vi "test_se_main_sid.vi"() -> ()   [LabVIEW 2016]
uses:
  <vilib>/rvi/DesktopExecutionNode/Execution/niFpgaDEN_Execute.vi
  <vilib>/rvi/DesktopExecutionNode/DesktopExecutionNode.xnode
panel:
  in  "se.sid.idParams":T1
  out "prbsSignal":T2(array[cluster])
  out "positionGraph":dbl[][](graph)
  out "positionGraph 2":dbl[][](graph)
  in  "scanTurnOnTime":i32=500
  out "itcSIDOutput":bool[](array[boolean])
  out "sidRepetition":u16[](array[numeric])
  out "sidRunning":bool[](array[boolean])
  out "positionSID":T3(array[cluster]) {"outputInt"."x" format="%.17g"; "outputInt"."y" format="%.17g"}
  out "position":T4(array[cluster]) {"outputInt"."x" format="%.16g"; "outputInt"."y" format="%.16g"}
  in  "se.sid.axisXnotY":bool=TRUE
  in  "sidOnTime":i32=6000
  in  "se.p.clocks":T5={"outputRate"=4, "fastDecFactor"=0, "outWaveSizeFast"=128, "pplUpsampling"=0, "numLines"=16, "se.p.fastInvDec"=0.0, "se.p.slowUpStep"=0.0, "se.p.outWaveSizeSlow"=128, "blankingMax"=6000000, "se.p.fastBlanking"={"startFwd"=0, "endFwd"=0, "startBwd"=0, "endBwd"=0, "disableBlanking"=TRUE, "useCoarseCounter"=FALSE}}
  in  "se.mot.p.target":cluster{"x":fxp<+/-,16,1>, "y":fxp<+/-,16,1>}[](array[cluster])=[{"x"=0.20001220703125, "y"=0.20001220703125}]
  in  "outputParams":T6={"se.p.scanOffsets"={"x"=0.0, "y"=0.0}, "se.p.transformMatrix"={"a"=1.0, "b"=0.0, "c"=0.0, "d"=1.0}, "se.p.scanSize"={"fastScanSize"=0.399993896484375, "slowScanSize"=0.399993896484375, "invertSlowAxis"=FALSE}}
  in  "se.p.modes":T7
  in  "se.mot.p.clocks":T8={"moveToDecFactor"=9, "moveToWaveSize"=128, "se.mot.p.invDec"=0.0}
  out "simulationProgressDone":dbl(slide)=0.9999166666666667 scale=0.0..1.0
  in  "simulationTime (ticks)":i32=12000
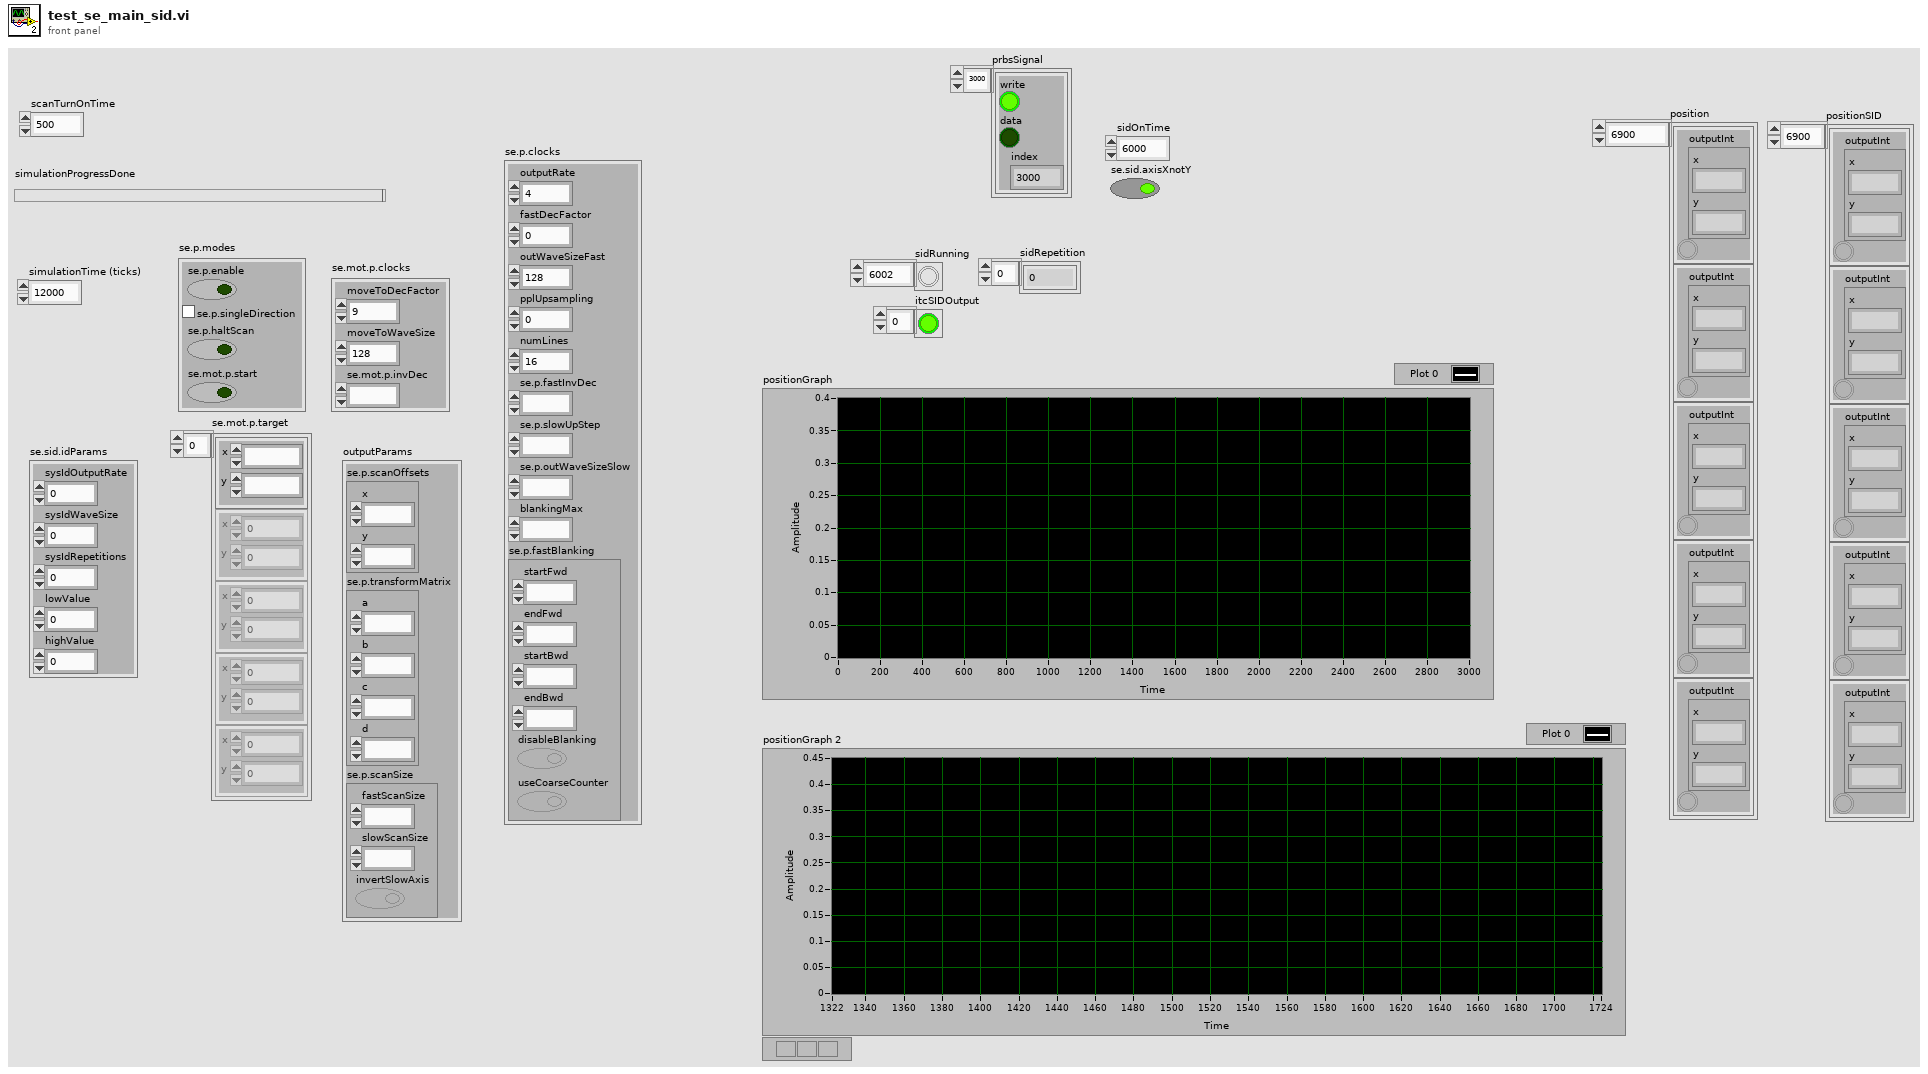
[diagram p1: front panel]
types:
  T1 = cluster{"sysIdOutputRate":u16, "sysIdWaveSize":u16, "sysIdRepetitions":u16, "lowValue":fxp<+/-,16,1>, "highValue":fxp<+/-,16,1>}
  T2 = cluster{"write":bool, "data":bool, "index":u16}[]
  T3 = cluster{"outputInt":cluster{"sid.o.height":fxp<+/-,28,1>, "sid.o.height":fxp<+/-,28,1>}, bool}[]
  T4 = cluster{"outputInt":cluster{"y":fxp<+/-,16,1>, "y":fxp<+/-,16,1>}, bool}[]
  T5 = cluster{"outputRate":u16, "fastDecFactor":u16, "outWaveSizeFast":u16, "pplUpsampling":u16, "numLines":u16, "se.p.fastInvDec":fxp<+,22,0>, "se.p.slowUpStep":fxp<+,28,0>, "se.p.outWaveSizeSlow":u16, "blankingMax":u32, "se.p.fastBlanking":cluster{"startFwd":u32, "endFwd":u32, "startBwd":u32, "endBwd":u32, "disableBlanking":bool, "useCoarseCounter":bool}}
  T6 = cluster{"se.p.scanOffsets":cluster{"x":fxp<+/-,16,1>, "y":fxp<+/-,16,1>}, "se.p.transformMatrix":cluster{"a":fxp<+/-,18,2>, "b":fxp<+/-,18,2>, "c":fxp<+/-,18,2>, "d":fxp<+/-,18,2>}, "se.p.scanSize":cluster{"fastScanSize":fxp<+,17,1>, "slowScanSize":fxp<+,17,1>, "invertSlowAxis":bool}}
  T7 = cluster{"se.p.enable":bool, "se.p.singleDirection":bool, "se.p.haltScan":bool, "se.mot.p.start":bool}
  T8 = cluster{"moveToDecFactor":u16, "moveToWaveSize":u16, "se.mot.p.invDec":fxp<+,16,0>}
  T9 = cluster{"a":fxp<+/-,18,2>, "b":fxp<+/-,18,2>, "c":fxp<+/-,18,2>, "d":fxp<+/-,18,2>}
  T10 = cluster{"fastScanSize":fxp<+,17,1>, "slowScanSize":fxp<+,17,1>, "invertSlowAxis":bool}
  T11 = cluster{"outputInt":cluster{"y":fxp<+/-,16,1>, "y":fxp<+/-,16,1>}, bool}
  T12 = cluster{"outputInt":cluster{"sid.o.height":fxp<+/-,28,1>, "sid.o.height":fxp<+/-,28,1>}, bool}
  T13 = cluster{"sid.o.height":fxp<+/-,28,1>, "sid.o.height":fxp<+/-,28,1>}
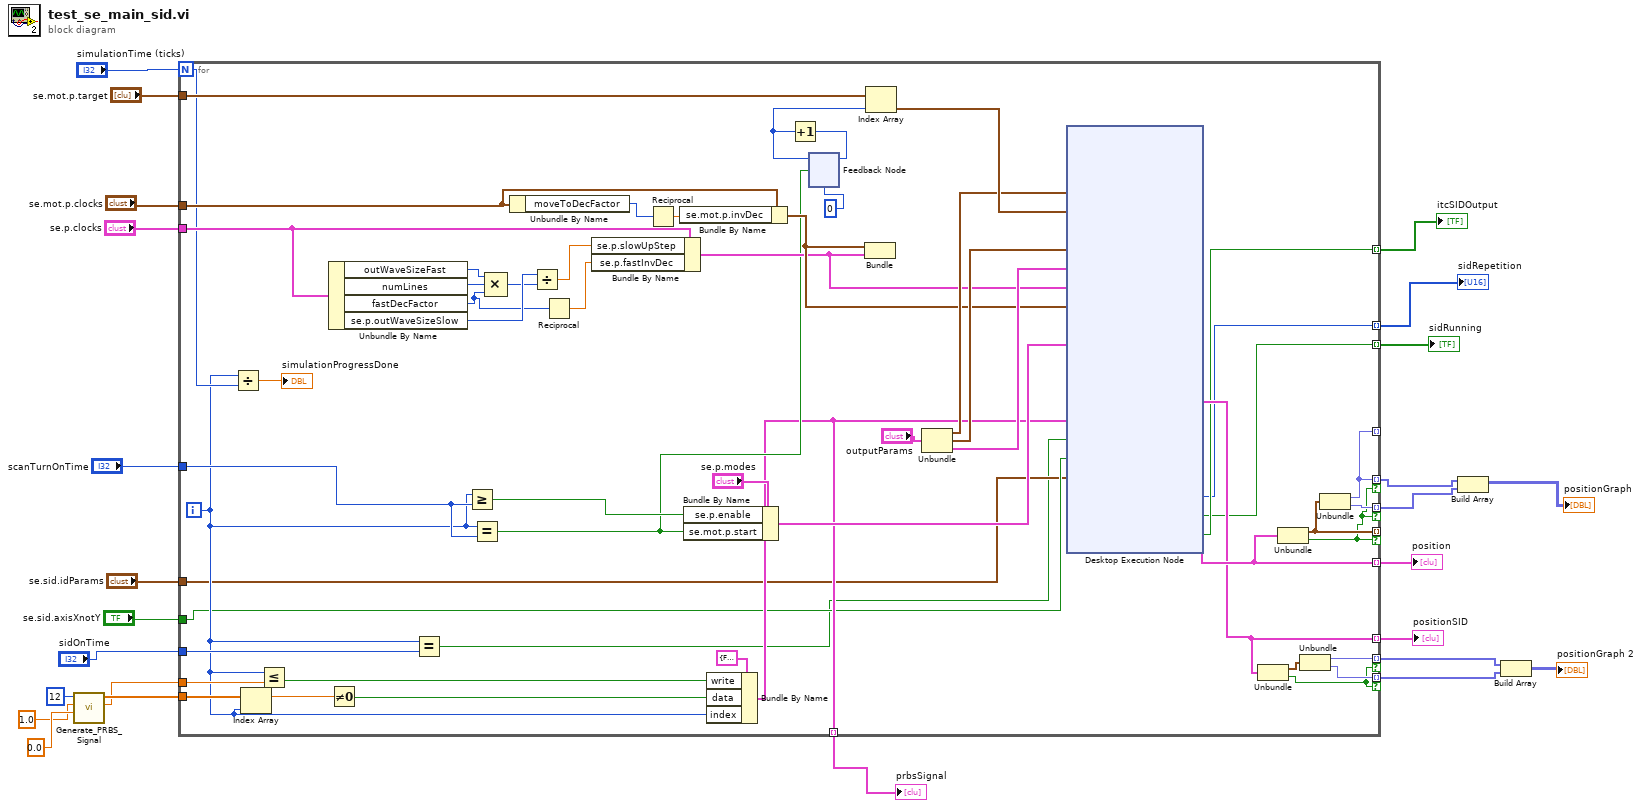
[diagram p0: block diagram]
diagram:
  n1 = call "Generate_PRBS_Signal.vi"("Min.Value"=0.0, "Max. Value"=1.0, "PRBS Order"=12) -> ("PRBS Signal Length"=w5:dbl, "PRBS Signal"=w6:dbl[])  [unwired: 7 in]
  n2 = for {
    N: "simulationTime (ticks)" -> [w64]
    tunnel: "se.mot.p.clocks" -> [w68]
    tunnel: "se.p.clocks" -> [w67]
    tunnel: "se.mot.p.target" -> [w66]
    tunnel: "se.sid.idParams" -> [w30]
    tunnel: "sidOnTime" -> [w52]
    tunnel: "se.sid.axisXnotY" -> [w31]
    tunnel: [w44] -> w19 mode=indexing
    tunnel: [w51] -> w18 mode=indexing
    tunnel: [w26] -> w17 mode=indexing
    tunnel: [w27] -> w16 mode=indexing
    tunnel: [w28] -> w15 mode=indexing
    tunnel: [w50] -> _ mode=indexing if=w48
    tunnel: [w45] -> w14 mode=indexing if=w48
    tunnel: [w49] -> w13 mode=indexing if=w48
    tunnel: "scanTurnOnTime" -> [w47]
    tunnel: [w45] -> _ mode=indexing
    tunnel: [w42] -> w11 mode=indexing if=w40
    tunnel: [w41] -> w10 mode=indexing if=w40
    tunnel: w6 -> [w39]
    tunnel: w5 -> [w38]
    tunnel: [w32] -> w2 mode=indexing
    i -> [w33]
    n3 = Divide(x=w33, y=w64) -> (x/y=→"simulationProgressDone":dbl)
    n4 = Index Array(array=w39, index=w33) -> (element=w34:dbl)
    n5 = Less Or Equal?(x=w33, y=w38) -> (x <= y?=w35:bool)
    n6 = Unbundle By Name(w67) -> ("outWaveSizeFast"=w74:u16, "numLines"=w75:u16, "fastDecFactor"=w70:u16, "se.p.outWaveSizeSlow"=w73:u16)
    n7 = Not Equal To 0?(x=w34) -> (x != 0?=w36:bool)
    n8 = Equal?(x=w33, y=w52) -> (x = y?=w29:bool)
    n9 = Greater Or Equal?(x=w33, y=w47) -> (x >= y?=w65:bool)
    n10 = Equal?(x=w33, y=w47) -> (x = y?=w46:bool)
    n11 = Compound Arithmetic op=MULTIPLY(w74, w75, w70) -> (w72:u16)
    n12 = Unbundle By Name(w68) -> ("moveToDecFactor"=w77:u16)
    n13 = Divide(x=w73, y=w72) -> (x/y=w71:dbl)
    n14 = Reciprocal(x=w70) -> (1/x=w69:dbl)
    n15 = Bundle By Name(cluster=w67, "se.p.slowUpStep"=w71, "se.p.fastInvDec"=w69) -> (w53:T5)
    n16 = Reciprocal(x=w77) -> (1/x=w76:dbl)
    n17 = Bundle By Name(cluster=w68, "se.mot.p.invDec"=w76) -> (w54:T8)
    n18 = Bundle By Name(cluster="se.p.modes", "se.p.enable"=w65, "se.mot.p.start"=w46) -> (w59:T7)
    n19 = Bundle By Name(cluster=cluster{"write":bool, "data":bool, "index":u16} {"write"=FALSE, "data"=FALSE, "index"=0} ("se.sid.m.sequence"), "write"=w35, "data"=w36, "index"=w33) -> (w32:cluster{"write":bool, "data":bool, "index":u16})
    n20 = feedback #1(0) -> (w62:i32)
    n21 = Increment(x=w62) -> (x+1=w61:i32)
    n22 = feedback-in #1(w61, w46) -> ()
    n23 = Bundle("se.mot.p.clocks"=w54, "se.p.clocks"=w53) -> ()  [unwired: 1 in, 1 out]
    n24 = Index Array(array=w66, index=w62) -> (element=w60:cluster{"x":fxp<+/-,16,1>, "y":fxp<+/-,16,1>})
    n25 = Unbundle("outputParams") -> ("se.p.scanOffsets"=w55:cluster{"x":fxp<+/-,16,1>, "y":fxp<+/-,16,1>}, "se.p.transformMatrix"=w56:T9, "se.p.scanSize"=w57:T10)
    n26 = xnode "Desktop Execution Node"("se.p.scanOffsets"=w55, "se.mot.p.target"=w60, "se.p.transformMatrix"=w56, "se.p.scanSize"=w57, "se.p.clocks"=w53, "se.mot.p.clocks"=w54, "se.p.modes"=w59, "se.sid.m.sequence"=w32, "se.sid.start"=w29, "se.sid.p.axisXNotY"=w31, "se.sid.p.params"=w30) -> ("se.o.position"=w51:T11, "se.o.positionSID"=w44:T12, "se.sid.s.repetitions"=w27:u16, "se.sid.s.running"=w26:bool, "se.sid.itcOutput"=w28:bool)  [unwired: 1 in, 4 out]
    n27 = Unbundle(w44) -> ("outputInt"=w43:T13, w40:bool)
    n28 = Unbundle(w51) -> ("outputInt"=w50:cluster{"y":fxp<+/-,16,1>, "y":fxp<+/-,16,1>}, w48:bool)
    n29 = Unbundle(w43) -> ("sid.o.height"=w42:fxp<+/-,28,1>, "sid.o.height"=w41:fxp<+/-,28,1>)
    n30 = Unbundle(w50) -> ("y"=w45:fxp<+/-,16,1>, "y"=w49:fxp<+/-,16,1>)
  }
  "position" <- w18
  "positionSID" <- w19
  "sidRunning" <- w17
  "sidRepetition" <- w16
  "itcSIDOutput" <- w15
  "prbsSignal" <- w2
  n31 = Build Array(w14, w13) -> (→"positionGraph":fxp<+/-,16,1>[][])
  n32 = Build Array(w11, w10) -> (→"positionGraph 2":fxp<+/-,28,1>[][])
